vi "Slow Move.vi"(8 "error in (no error)":errorcluster, 11 "SwipeScrollListbox in":refnum<class "SwipeScrollListbox.lvclass">) -> (0 "error out":errorcluster, 3 "SwipeScrollListbox out":refnum<class "SwipeScrollListbox.lvclass">)   [LabVIEW 2019, in "SwipeScrollListbox.lvclass"]
uses:
  SwipeScrollListbox.lvclass
  SwipeScrollListbox.lvclass/SwipeScrollListbox.ctl
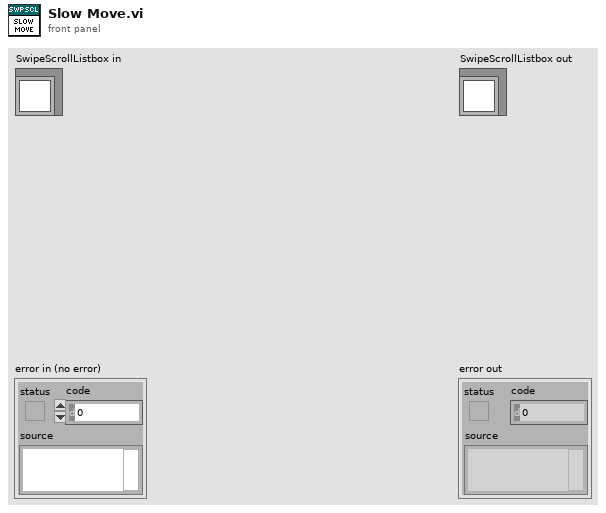
[diagram p1: front panel]
types:
  T1 = typedef "SwipeScrollListbox.lvclass/State Data.ctl" = cluster{"Timeout":i32, "Time":timestamp, "Y":i32, "Slow Distance":i32, "Rate":dbl, "Row Selected":i32}
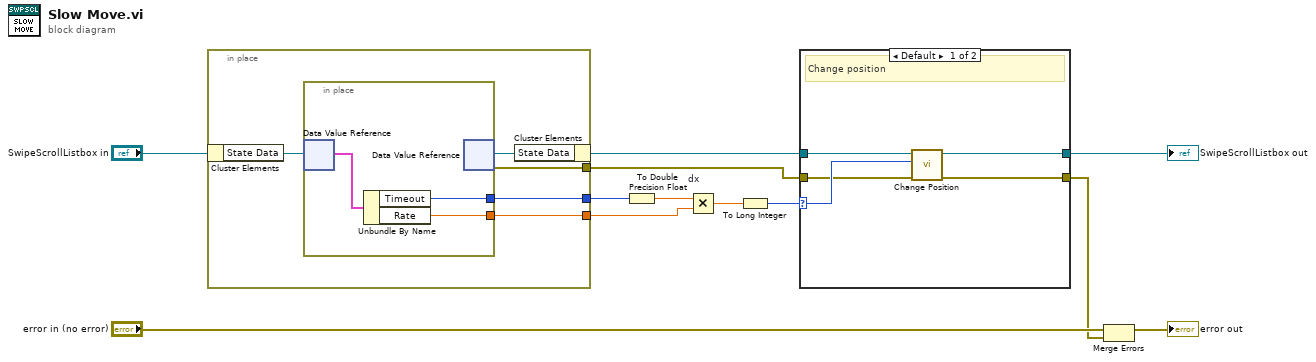
[diagram p0: block diagram]
diagram:
  n1 = in-place {
    in-place-border: [w16] -> w9
    in-place-border: [w14] -> w8
    in-place-border: [w13] -> w4
    n2 = in-place-cluster #1("SwipeScrollListbox in") -> ("State Data"=w17:refnum<data-value>)
    n3 = in-place {
      in-place-border: [w19] -> w16
      in-place-border: [w18] -> w14
      n4 = in-place-dvr #2(w17) -> (w20:T1)  [unwired: 1 out]
      n5 = Unbundle By Name(w20) -> ("Timeout"=w19:i32, "Rate"=w18:dbl)
      n6 = in-place-dvr #2() -> (w15:refnum<data-value>, w13:errorcluster)  [unwired: 1 in]
    }
    n7 = in-place-cluster #1("State Data"=w15) -> (w6:refnum<class "SwipeScrollListbox.lvclass">)
  }
  n8 = To Double Precision Float(number=w9) -> (double precision float=w11:dbl)
  n9 = Multiply "dx"(x=w11, y=w8) -> (x*y=w10:dbl)
  n10 = To Long Integer(number=w10) -> (32bit integer=w7:i32)
  n11 = case shown="Default" w7 {
    selector: w7 -> [w24 _]
    tunnel: w6 -> [w25 w27]
    tunnel: [w22 w27] -> w5
    tunnel: w4 -> [w23 w26]
    tunnel: [w21 w26] -> w1
    frame Default {
      # "Change position"
      n12 = call "Change Position.vi"("error in (no error)"=w23, "Position Change"=w24, "SwipeScrollListbox in"=w25) -> ("error out"=w21:errorcluster, "SwipeScrollListbox out"=w22:refnum<class "SwipeScrollListbox.lvclass">)  [unwired: 7 in]
    }
    frame -5..5 {
      # "Slow down and stop at item"
    }
  }
  "SwipeScrollListbox out" <- w5
  n13 = Merge Errors("error in (no error)", w1) -> (→"error out":errorcluster)
